vi "Unflatten Value.vi"(8 "Error In":errorcluster, 10 "Value":string, 11 "Int Array In":refnum<class "1D Int.lvclass">) -> (0 "Error Out":errorcluster, 3 "Int Array Out":refnum<class "1D Int.lvclass">)   [LabVIEW 2017, in "Tree API.lvlib" / "1D Int.lvclass"]
uses:
  1D Int.lvclass
  Tree Manager/Tree.lvclass
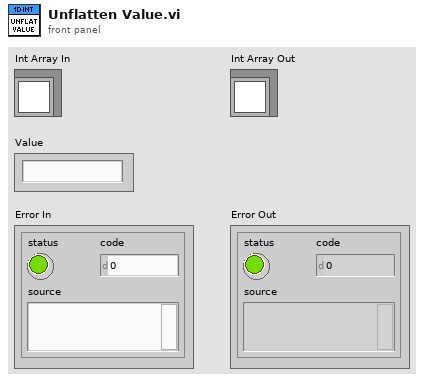
[diagram p1: front panel]
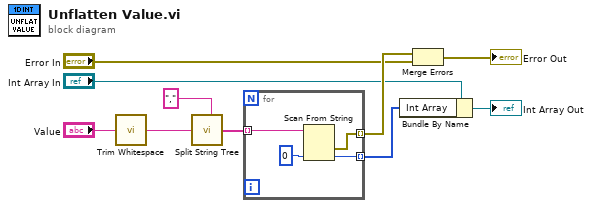
[diagram p0: block diagram]
diagram:
  n1 = call <vilib>:"Trim Whitespace.vi"("string"="Value") -> ("trimmed string"=w1:string)  [unwired: 1 in]
  n2 = call "Split String Tree.vi"("Split Pattern"="," ("Separator (,)"), "Input String"=w1) -> ("Split String"=w7:string[])  [unwired: 5 in]
  n3 = for {
    tunnel: [w13] -> w9 mode=indexing
    tunnel: [w12] -> w8 mode=indexing
    tunnel: w7 -> [w11] mode=indexing
    n4 = Scan From String(input string=w11, default 1=i64 0 ("default value 1")) -> (error out=w12:errorcluster, output 1=w13:i64)  [unwired: 3 in, 2 out]
  }
  n5 = Bundle By Name(cluster="Int Array In", "Int Array"=w9) -> (→"Int Array Out":refnum<class "1D Int.lvclass">)
  n6 = Merge Errors(w8, "Error In") -> (→"Error Out":errorcluster)
